vi "runDisplay.vi"(8 "error in (no error)":errorcluster, 11 "Display":refnum<class "DisplayBase.lvclass">) -> (0 "error out":errorcluster, 3 "Display":refnum<class "DisplayBase.lvclass">)   [LabVIEW 2020, in "DisplayBase.lvclass"]
uses:
  DisplayBase.lvclass
panel:
  # "Connector Pane"
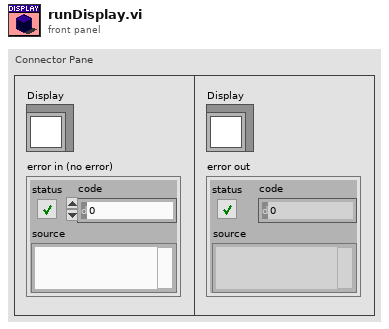
[diagram p1: front panel]
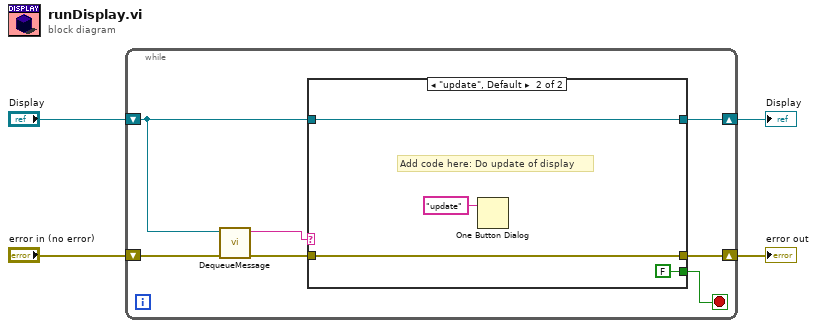
[diagram p0: block diagram]
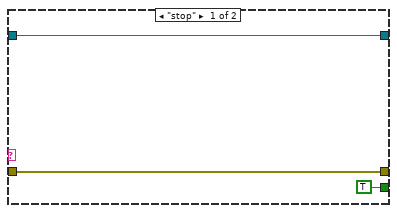
[diagram p2: hidden frame]
diagram:
  n1 = while {
    shift-right: [w8] -> w3
    shift-left: "error in (no error)" -> [w11]
    shift-right: [w7] -> w4
    shift-left: "Display" -> [w5]
    stop <- w6 stop-if-true
    n2 = call "DequeueMessage.vi"("error in (no error)"=w11, "DisplayBase in"=w5) -> ("error out"=w9:errorcluster, "String"=w10:string)  [unwired: 8 in]
    n3 = case shown="\"update\", Default" w10 {
      tunnel: w5 -> [w12 w17]
      tunnel: w9 -> [w14 w18]
      tunnel: [w14 w18] -> w8
      tunnel: [w12 w17] -> w7
      tunnel: [TRUE FALSE] -> w6
      frame "stop" {
      }
      frame "update", Default {
        # "Add code here: Do update of display"
        n4 = One Button Dialog(message="update") -> ()  [unwired: 1 in, 1 out]
      }
    }
  }
  "Display" <- w4
  "error out" <- w3
